vi "ReadDiagnosticInformation_ByStatus.vi"(8 "error in (no error)":errorcluster, 10 "status mask":T1, 11 "diag ref in":T2) -> (0 "error out":errorcluster, 1 "success?":bool, 2 "data out":u8[](array[numeric]), 3 "diag ref out":T2)   [LabVIEW 2013, in "GMLAN.lvlib"]
uses:
  GMLAN.lvlib
  <vilib>/Automotive Diagnostic Command Set/Diagnostic Transport.llb/Diag Reference.ctl
  <vilib>/Automotive Diagnostic Command Set/Diagnostic Transport.llb/Transport Protocol Selector.ctl
  <vilib>/Automotive Diagnostic Command Set/Diagnostic Transport.llb/Diag CAN Frame Log.ctl
  DTCStatusMask.ctl
  <vilib>/addons/Automotive Diagnostic Command Set/NI_Automotive Diagnostic Command Set.lvlib
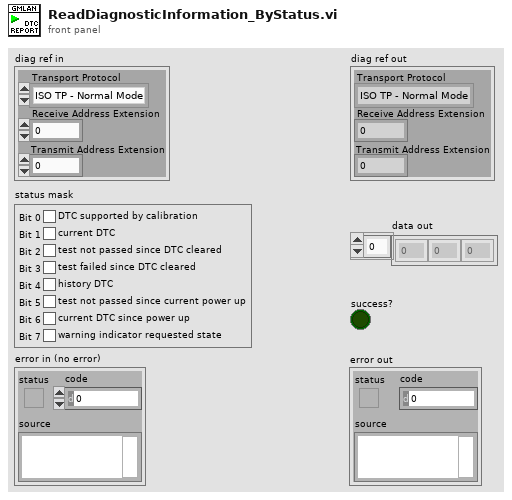
[diagram p1: front panel]
types:
  T1 = typedef "GMLAN.lvlib/DTCStatusMask.ctl" = cluster{"DTC supported by calibration":bool, "current DTC":bool, "test not passed since DTC cleared":bool, "test failed since DTC cleared":bool, "history DTC":bool, "test not passed since current power up":bool, "current DTC since power up":bool, "warning indicator requested state":bool}
  T2 = typedef "NI_Automotive Diagnostic Command Set.lvlib/Diag Reference.ctl" = cluster{"Diag CAN Handle":u32, "Transport Protocol":T3, "Receive Address Extension":u8, "Transmit Address Extension":u8, "Receive CAN Id":u32, "Transmit CAN Id":u32, "Diag CAN Queue":refnum<queue>, "Log Frames ?":bool, "My TP Address":u8, "Other TP Address":u8, "T1":u16, "T2":u16, "T3":u16, "T4":u16, "Tx SN":u8, "Block Size":u8, "Rx SN":u8, "VW TP Initialized?":bool, "Tx block no":u8, "baud rate":u32, "Interface":string, "Channel Diag CAN Handle":u32, "UDP Connection ID":refnum<k16>, "TCP Connection ID":refnum<k5>, "Target IP Addr":u32, "Source Address":u16, "Target Address":u16, "Send Header NACK?":bool, "DLL Handle":u32, "NAD":u8}
  T3 = typedef "NI_Automotive Diagnostic Command Set.lvlib/Transport Protocol Selector.ctl" = enum16{"ISO TP - Normal Mode", "ISO TP - Mixed Mode", "VW TP 2.0", "Diagnostics on IP", "ISO TP LIN"}
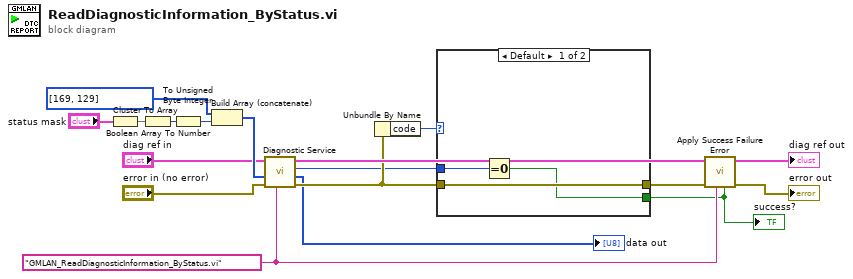
[diagram p0: block diagram]
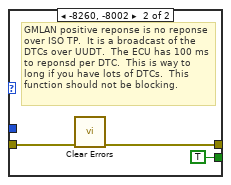
[diagram p2: hidden frame]
diagram:
  w8 = "GMLAN_ReadDiagnosticInformation_ByStatus.vi" ("error source")
  n1 = Cluster To Array(cluster="status mask") -> (array=w4:bool[])
  n2 = Boolean Array To Number(Boolean array=w4) -> (number=w2:u32)
  n3 = To Unsigned Byte Integer(number=w2) -> (unsigned 8bit integer=w1:u8)
  n4 = Build Array (concatenate)(u8[] [169, 129], w1) -> (w14:u8[])
  n5 = call <vilib>:"Diagnostic Service.vi"("error source"=w8, "error in (no error)"="error in (no error)", "data in"=w14, "diag ref in"="diag ref in") -> ("error out"=w15:errorcluster, "data out"=→"data out":u8[], "error code"=w11:u8, "diag ref out"=→"diag ref out":T2)  [unwired: 2 in, 2 out]
  n6 = Unbundle By Name(w15) -> ("code"=w7:i32)
  n7 = case shown="Default" w7 {
    tunnel: w15 -> [w20 w23]
    tunnel: [w20 w22] -> w6
    tunnel: w11 -> [w19 _]
    tunnel: [w18 TRUE] -> w5
    frame Default {
      n8 = Equal To 0?(x=w19) -> (x = 0?=w18:bool)
    }
    frame -8260, -8002 {
      # "GMLAN positive reponse is no reponse over ISO TP.  It is a broadcast of the DTCs over UUDT.  The ECU has 100 ms to reponsd per DTC.  This is way to long if you have lots of DTCs.  This function should not be blocking."
      n9 = call <vilib>:"Clear Errors.vi"("error in (no error)"=w23) -> ("error out"=w22:errorcluster)  [unwired: 6 in]
    }
  }
  "success?" <- w5
  n10 = call <vilib>:"Apply Success Failure Error.vi"("success code"=w5, "error source"=w8, "error in (no error)"=w6) -> ("error out"=→"error out":errorcluster)  [unwired: 8 out]
